vi "onStopped.vi"(8 "error in (no error)":errorcluster, 11 "SMO.ErrorInjection":refnum<class "SMO.ErrorInjection.lvclass">) -> (0 "error out":errorcluster, 3 "SMO.ErrorInjection out":refnum<class "SMO.ErrorInjection.lvclass">)   [LabVIEW 2013, in "SMO.ErrorInjection.lvclass"]
uses:
  SMO.ErrorInjection.lvclass
  src/SMO/SMO.lvclass
panel:
  # "For instructions on how to use the JKI State Machine Objects, examples and video tutorials, visit:\nhttp://jki.net/state-machine-objects/\n\nJKI State Machine Objects™\nhttp://jki.net/state-machine-objects/\nCopyright (C) 2005-2015, JKI <info@jki.net>\nALL RIGHTS RESERVED"
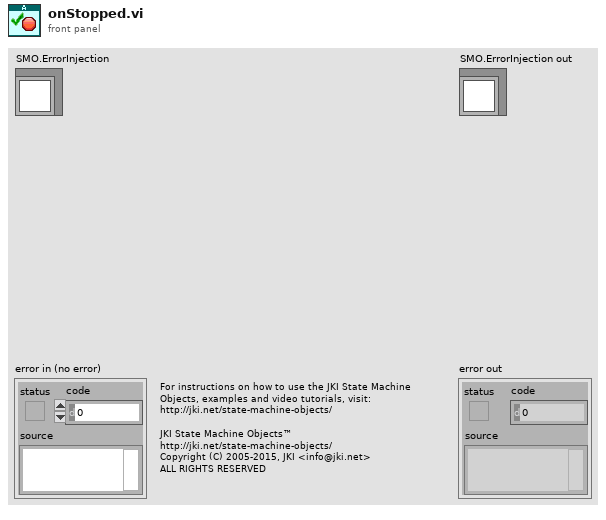
[diagram p1: front panel]
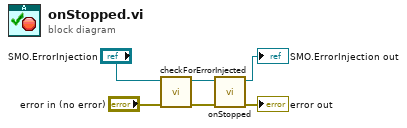
[diagram p0: block diagram]
diagram:
  n1 = call "checkForErrorInjected.vi"("error in (no error)"="error in (no error)", "SMO.ErrorInjection in"="SMO.ErrorInjection") -> ("error out"=w4:errorcluster, "SMO.ErrorInjection dup"=w1:refnum<class "SMO.ErrorInjection.lvclass">)  [unwired: 8 in]
  n2 = call-parent "onStopped.vi"("error in (no error)"=w4, "SMO"=w1) -> ("error out"=→"error out":errorcluster, "SMO out"=→"SMO.ErrorInjection out":refnum<class "SMO.ErrorInjection.lvclass">)  [unwired: 8 in]
